vi "SMC.vi"() -> ()   [LabVIEW 2009]
doc: "This is the Superconducting Magnet Control module (SMC).\nIts job is to receive messages from the PDP, translate them into magnet commands, and send reply messages back to the PDP indicating magnet status."
uses:
  SMC Global.vi
panel:
  in  "Read\nWitness?":bool
  in  "Force Read":bool
  in  "Need to Beep":bool
  in  "Beep at Setpoint":bool=TRUE
  out "SMC Message Type":T1(ring)=enum."Ping="
  out "Magnet Entered this state at:":string
  out "Last Change":dbl format="%.2f"
  out "Update Often":bool
  out "Magnet Status":T2={"Sweep Status"=enum."To Zero", "Leads Current (A)"=0.0, "Leads Voltage (V)"=0.0, "Leads Field (T)"=0.0, "Switch Heater"=FALSE, "Setpoint (A)"=0.0, "Sweep Rate (A/min)"=0.0, "System Status"=enum."Warming Up", "Limit Status"=enum."Positive Current Limit", "Persistent Current (A)"=0.0, "Control Status"=FALSE, "Persistent Field (T)"=0.0} {"Leads Field (T)" format="%.2f"; "Persistent Field (T)" format="%.3f"; "Persistent Current (A)" format="%.3f"; "Setpoint (A)" format="%.3f"; "Leads Voltage (V)" format="%.2f"; "Sweep Rate (A/min)" format="%.2f"; "Leads Current (A)" format="%.3f"}
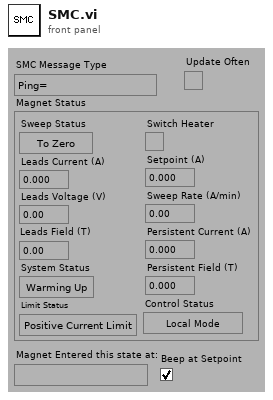
[diagram p1: front panel]
types:
  T1 = enum16{"Bad Message", "DoNothing", "Read=", "GenEvent=", "MagStatus=", "Control", "Setpoint=", "Setrate=", "Heater=", "Ping=", "Stop", "Beep"}
  T2 = cluster{"Sweep Status":enum16{"Hold", "To Setpoint", "To Zero", "Clamped"}, "Leads Current (A)":dbl, "Leads Voltage (V)":dbl, "Leads Field (T)":dbl, "Switch Heater":bool, "Setpoint (A)":dbl, "Sweep Rate (A/min)":dbl, "System Status":enum16{"Normal", "Quenched", "Over Heated", "Warming Up"}, "Limit Status":enum16{"Normal", "Positive Voltage Limit", "Negative Voltage Limit", "Negative Current Limit", "Positive Current Limit"}, "Persistent Current (A)":dbl, "Control Status":bool, "Persistent Field (T)":dbl}
  T3 = enum16{"Hold", "To Setpoint", "To Zero", "Clamped"}
  T4 = enum16{"Normal", "Quenched", "Over Heated", "Warming Up"}
  T5 = enum16{"Normal", "Positive Voltage Limit", "Negative Voltage Limit", "Negative Current Limit", "Positive Current Limit"}
  T6 = cluster{"Sweep Status":enum16{"Hold", "To Setpoint", "To Zero", "Clamped"}, "Leads Current (A)":dbl, "Leads Field (T)":dbl, "Switch Heater":bool, "Setpoint (A)":dbl, "Sweep Rate (A/min)":dbl, "System Status":enum16{"Normal", "Quenched", "Over Heated", "Warming Up"}, "Limit Status":enum16{"Normal", "Positive Voltage Limit", "Negative Voltage Limit", "Negative Current Limit", "Positive Current Limit"}, "Persistent Current (A)":dbl, "Control Status":bool, "Persistent Field (T)":dbl}
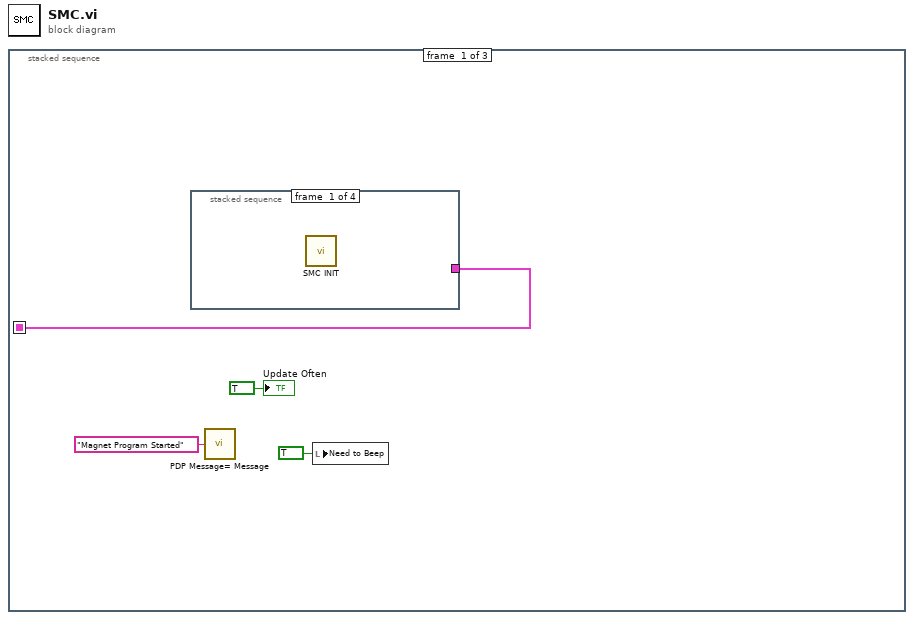
[diagram p0: block diagram]
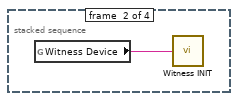
[diagram p2: hidden frame]
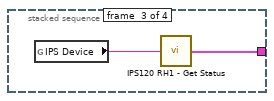
[diagram p3: hidden frame]
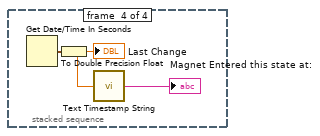
[diagram p4: hidden frame]
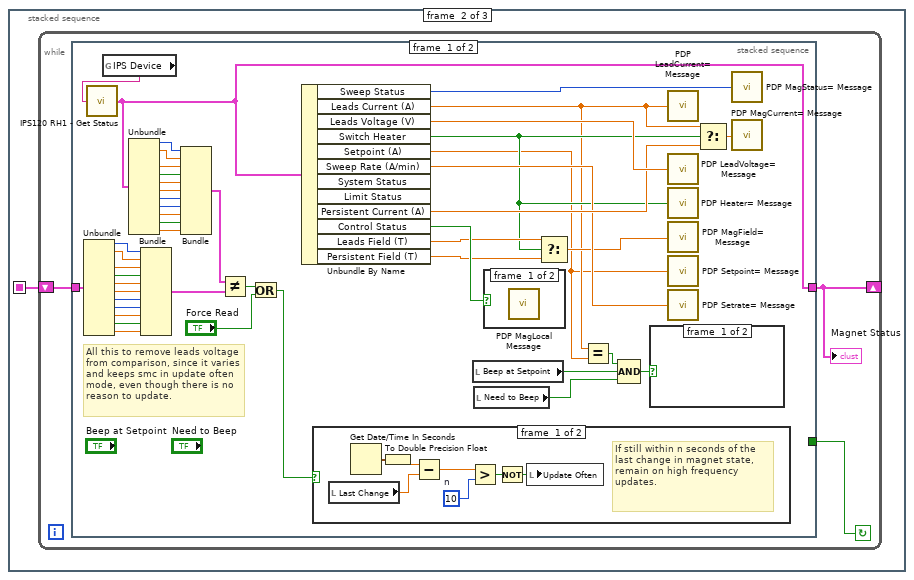
[diagram p5: hidden frame]
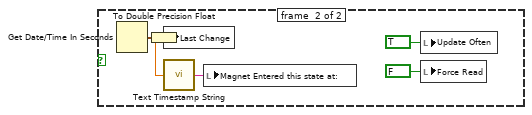
[diagram p6: hidden frame]
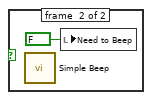
[diagram p7: hidden frame]
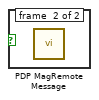
[diagram p8: hidden frame]
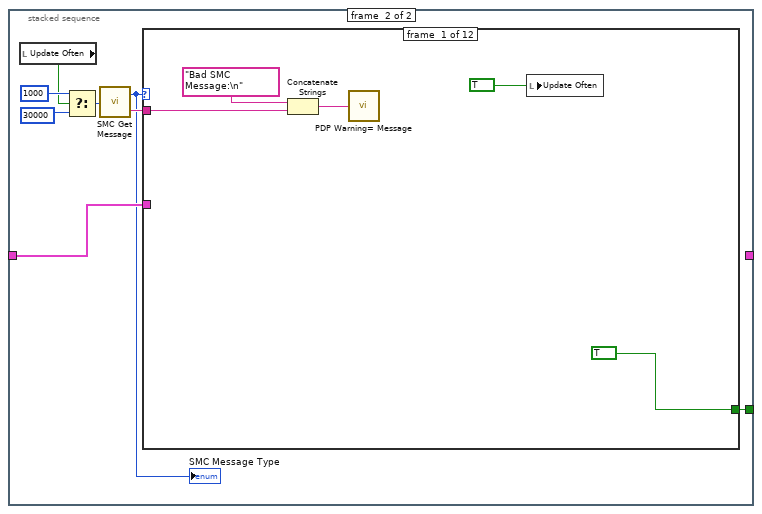
[diagram p9: hidden frame]
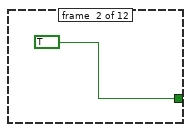
[diagram p10: hidden frame]
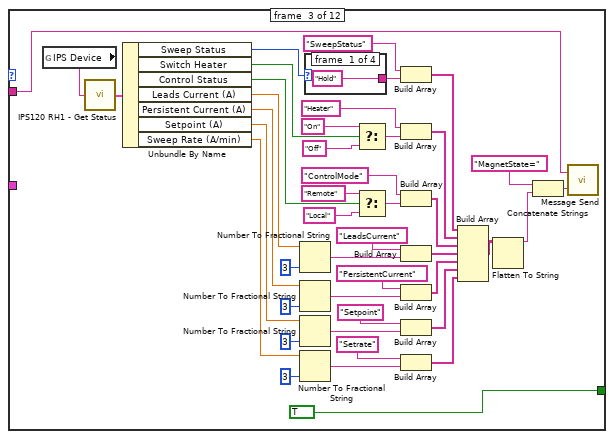
[diagram p11: hidden frame]
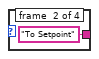
[diagram p12: hidden frame]
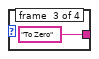
[diagram p13: hidden frame]
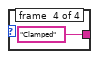
[diagram p14: hidden frame]
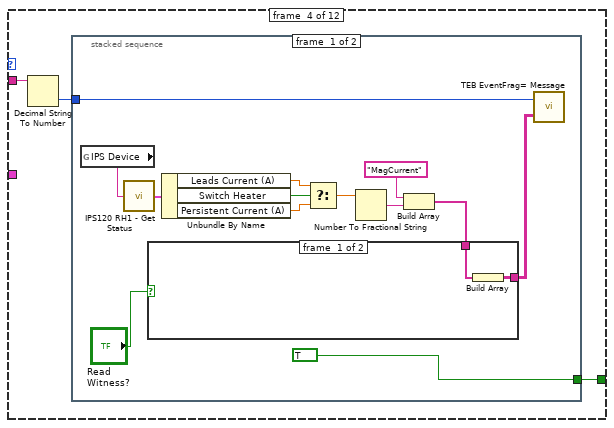
[diagram p15: hidden frame]
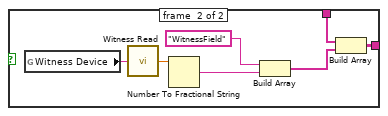
[diagram p16: hidden frame]
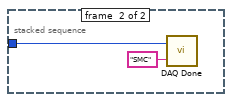
[diagram p17: hidden frame]
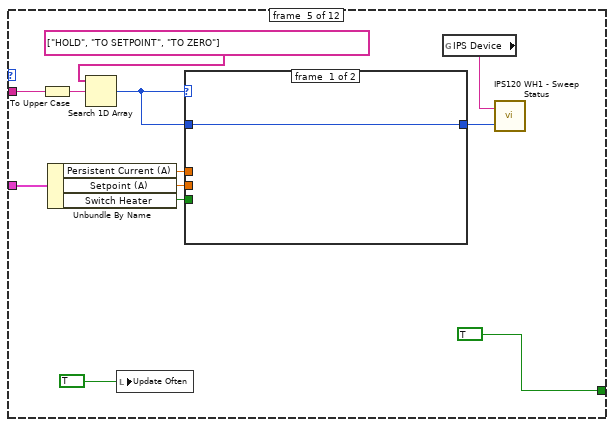
[diagram p18: hidden frame]
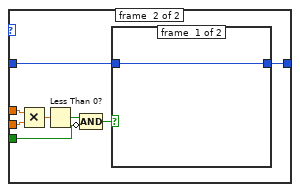
[diagram p19: hidden frame]
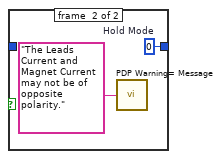
[diagram p20: hidden frame]
diagram:
  n1 = stacked-sequence {
    seq-local: [w4 _ _] -> [_ w11 _]
    frame #0 {
      n2 = stacked-sequence {
        tunnel: [_ _ w7 _] -> w4
        frame #0 {
          n3 = call "SMC INIT.vi"() -> ()  [unwired: 1 in]
        }
        frame #1 {
          n4 = global read "SMC Global.vi" "Witness Device"() -> (w5:string)
          n5 = call "Witness INIT.vi"("address string"=w5) -> ()
        }
        frame #2 {
          n6 = global read "SMC Global.vi" "IPS Device"() -> (w6:string)
          n7 = call "IPS120 RH1 - Get Status.vi"("GPIB Address"=w6) -> ("Magnet Status"=w7:T2)
        }
        frame #3 {
          n8 = Get Date/Time In Seconds() -> (seconds since 1Jan1904=w8:timestamp)
          n9 = To Double Precision Float(number=w8) -> (double precision float=w10:dbl)
          "Last Change" <- w10
          n10 = call "Text Timestamp String.vi"("Seconds"=w10) -> ("Timestamp String"=→"Magnet Entered this state at:":string)
        }
      }
      n11 = call "PDP Message= Message.vi"("Message"="Magnet Program Started") -> ()
      n12 = local write "Need to Beep"(TRUE ("Need to Beep")) -> ()
      "Update Often" <- TRUE ("Update Often")
    }
    frame #1 {
      n13 = while {
        shift-left: w11 -> [w13]
        shift-right: [w12] -> _
        stop <- w14 continue-if-true
        n14 = stacked-sequence {
          tunnel: [_ w80] -> w14
          tunnel: w13 -> [w59 w76]
          tunnel: [w45 _] -> w12
          frame #0 {
            # "All this to remove leads voltage from comparison, since it varies and keeps smc in update often mode, even though there is no \nreason to update."
            n15 = Unbundle(w59) -> ("Sweep Status"=w58:T3, "Leads Current (A)"=w57:dbl, "Leads Field (T)"=w56:dbl, "Switch Heater"=w55:bool, "Setpoint (A)"=w54:dbl, "Sweep Rate (A/min)"=w53:dbl, "System Status"=w52:T4, "Limit Status"=w51:T5, "Persistent Current (A)"=w42:dbl, "Control Status"=w41:bool, "Persistent Field (T)"=w40:dbl)  [unwired: 1 out]
            n16 = global read "SMC Global.vi" "IPS Device"() -> (w60:string)
            n17 = call "IPS120 RH1 - Get Status.vi"("GPIB Address"=w60) -> ("Magnet Status"=w45:T2)
            n18 = Unbundle(w45) -> ("Sweep Status"=w34:T3, "Leads Current (A)"=w35:dbl, "Leads Field (T)"=w36:dbl, "Switch Heater"=w37:bool, "Setpoint (A)"=w38:dbl, "Sweep Rate (A/min)"=w39:dbl, "System Status"=w50:T4, "Limit Status"=w49:T5, "Persistent Current (A)"=w48:dbl, "Control Status"=w47:bool, "Persistent Field (T)"=w46:dbl)  [unwired: 1 out]
            n19 = Bundle("Sweep Status"=w58, "Leads Current (A)"=w57, "Leads Field (T)"=w56, "Switch Heater"=w55, "Setpoint (A)"=w54, "Sweep Rate (A/min)"=w53, "System Status"=w52, "Limit Status"=w51, "Persistent Current (A)"=w42, "Control Status"=w41, "Persistent Field (T)"=w40) -> (w43:T6)  [unwired: 1 in]
            n20 = Bundle("Sweep Status"=w34, "Leads Current (A)"=w35, "Leads Field (T)"=w36, "Switch Heater"=w37, "Setpoint (A)"=w38, "Sweep Rate (A/min)"=w39, "System Status"=w50, "Limit Status"=w49, "Persistent Current (A)"=w48, "Control Status"=w47, "Persistent Field (T)"=w46) -> (w44:T6)  [unwired: 1 in]
            n21 = Not Equal?(x=w44, y=w43) -> (x != y?=w32:bool)
            n22 = Or(x=w32, y="Force Read") -> (x .or. y?=w15:bool)
            n23 = Unbundle By Name(w45) -> ("Sweep Status"=w31:T3, "Leads Current (A)"=w21:dbl, "Leads Voltage (V)"=w30:dbl, "Switch Heater"=w23:bool, "Setpoint (A)"=w20:dbl, "Sweep Rate (A/min)"=w27:dbl, "Persistent Current (A)"=w29:dbl, "Control Status"=w26:bool, "Leads Field (T)"=w25:dbl, "Persistent Field (T)"=w24:dbl)  [unwired: 2 out]
            n24 = case shown="False" w15 {
              frame #0 {
                w64 = 10  # n
                # "If still within n seconds of the last change in magnet state, remain on high frequency updates."
                n25 = local read "Last Change"() -> (w63:dbl)
                n26 = Get Date/Time In Seconds() -> (seconds since 1Jan1904=w61:timestamp)
                n27 = To Double Precision Float(number=w61) -> (double precision float=w62:dbl)
                n28 = Subtract(x=w62, y=w63) -> (x-y=w65:dbl)
                n29 = Greater?(x=w65, y=w64) -> (0:w66:bool)
                n30 = Not(x=w66) -> (.not. x?=w67:bool)
                n31 = local write "Update Often"(w67) -> ()
              }
              frame #1 {
                n32 = Get Date/Time In Seconds() -> (seconds since 1Jan1904=w68:timestamp)
                n33 = To Double Precision Float(number=w68) -> (double precision float=w71:dbl)
                n34 = local write "Last Change"(w71) -> ()
                n35 = call "Text Timestamp String.vi"("Seconds"=w71) -> ("Timestamp String"=w72:string)
                n36 = local write "Magnet Entered this state at:"(w72) -> ()
                n37 = local write "Update Often"(TRUE ("Update Often")) -> ()
                n38 = local write "Force Read"(FALSE ("Force Read")) -> ()
              }
            }
            n39 = local read "Beep at Setpoint"() -> (w18:bool)
            n40 = local read "Need to Beep"() -> (w17:bool)
            n41 = case shown="False" w26 {
              frame #0 {
                n42 = call "PDP MagLocal Message.vi"() -> ()  [unwired: 1 in]
              }
              frame #1 {
                n43 = call "PDP MagRemote Message.vi"() -> ()  [unwired: 1 in]
              }
            }
            n44 = Select(t=w25, s=w23, f=w24) -> (s? t:f=w22:dbl)
            n45 = Equal?(x=w21, y=w20) -> (x = y?=w19:bool)
            n46 = Compound Arithmetic op=AND(w19, w18, w17) -> (w16:bool)
            n47 = case shown="True" w16 {
              frame #0 {
              }
              frame #1 {
                n48 = call "Simple Beep.vi"() -> ()  [unwired: 1 in]
                n49 = local write "Need to Beep"(FALSE) -> ()
              }
            }
            n50 = call "PDP LeadCurrent= Message.vi"("Lead Current"=w21) -> ()
            n51 = call "PDP LeadVoltage= Message.vi"("Lead Voltage"=w30) -> ()
            n52 = call "PDP Heater= Message.vi"("Setrate"=w23) -> ()
            n53 = call "PDP MagField= Message.vi"("Mag Field"=w22) -> ()
            n54 = call "PDP Setpoint= Message.vi"("Setpoint"=w20) -> ()
            n55 = call "PDP Setrate= Message.vi"("Setrate"=w27) -> ()
            n56 = Select(t=w21, s=w23, f=w29) -> (s? t:f=w28:dbl)
            n57 = call "PDP MagStatus= Message.vi"("Mag Status"=w31) -> ()
            n58 = call "PDP MagCurrent= Message.vi"("Mag Current"=w28) -> ()
          }
          frame #1 {
            n59 = local read "Update Often"() -> (w74:bool)
            n60 = Select(t=1000, s=w74, f=30000) -> (s? t:f=w79:i32)
            n61 = call "SMC Get Message.vi"("Timeout (ms)"=w79) -> ("SMC Message Type"=w75:T1, "Text"=w81:string)
            "SMC Message Type" <- w75
            n62 = case shown="\"Heater=\"" w75 {
              tunnel: w81 -> [w86 _ w91 w137 w173 _ w195 w200 w204 w248 _ _]
              tunnel: [TRUE TRUE TRUE w138 TRUE TRUE TRUE TRUE TRUE TRUE FALSE TRUE] -> w80
              tunnel: w76 -> [_ _ _ _ w166 w190 _ _ _ _ _ _]
              frame #0 {
                n63 = Concatenate Strings("Bad SMC Message:\n", w86) -> (w84:string)
                n64 = call "PDP Warning= Message.vi"("Message"=w84) -> ()
                n65 = local write "Update Often"(TRUE) -> ()
              }
              frame #1 {
              }
              frame #2 {
                n66 = global read "SMC Global.vi" "IPS Device"() -> (w130:string)
                n67 = call "IPS120 RH1 - Get Status.vi"("GPIB Address"=w130) -> ("Magnet Status"=w129:T2)
                n68 = Unbundle By Name(w129) -> ("Sweep Status"=w109:T3, "Switch Heater"=w110:bool, "Control Status"=w106:bool, "Leads Current (A)"=w121:dbl, "Persistent Current (A)"=w122:dbl, "Setpoint (A)"=w123:dbl, "Sweep Rate (A/min)"=w124:dbl)
                n69 = Number To Fractional String(number=w121, precision (6)=i16 3) -> (F-format string=w120:string)  [unwired: 2 in]
                n70 = Number To Fractional String(number=w122, precision (6)=i16 3) -> (F-format string=w118:string)  [unwired: 2 in]
                n71 = Number To Fractional String(number=w123, precision (6)=i16 3) -> (F-format string=w117:string)  [unwired: 2 in]
                n72 = Number To Fractional String(number=w124, precision (6)=i16 3) -> (F-format string=w116:string)  [unwired: 2 in]
                n73 = case shown="\"Hold\"" w109 {
                  tunnel: ["Hold" "To Setpoint" "To Zero" "Clamped"] -> w101
                  frame #0 {
                  }
                  frame #1 {
                  }
                  frame #2 {
                  }
                  frame #3 {
                  }
                }
                n74 = Select(t="On", s=w110, f="Off") -> (s? t:f=w104:string)
                n75 = Select(t="Remote", s=w106, f="Local") -> (s? t:f=w105:string)
                n76 = Build Array("SweepStatus", w101) -> (w95:string[])
                n77 = Build Array("Heater", w104) -> (w94:string[])
                n78 = Build Array("ControlMode", w105) -> (w93:string[])
                n79 = Build Array("LeadsCurrent", w120) -> (w96:string[])
                n80 = Build Array("PersistentCurrent", w118) -> (w97:string[])
                n81 = Build Array("Setpoint", w117) -> (w98:string[])
                n82 = Build Array("Setrate", w116) -> (w99:string[])
                n83 = Build Array(w95, w94, w93, w96, w97, w98, w99) -> (w92:string[][])
                n84 = Flatten To String(anything=w92) -> (data string=w89:string)  [unwired: 3 in, 2 out]
                n85 = Concatenate Strings("MagnetState=" ("Substring"), w89) -> (w90:string)
                n86 = call "Message Send.vi"("Message"=w90, "Destination"=w91) -> ()
              }
              frame #3 {
                n87 = Decimal String To Number(string=w137) -> (number=w136:i32)  [unwired: 2 in, 1 out]
                n88 = stacked-sequence {
                  tunnel: [TRUE _] -> w138
                  tunnel: w136 -> [w150 w162]
                  frame #0 {
                    n89 = global read "SMC Global.vi" "IPS Device"() -> (w144:string)
                    n90 = call "IPS120 RH1 - Get Status.vi"("GPIB Address"=w144) -> ("Magnet Status"=w149:T2)
                    n91 = Unbundle By Name(w149) -> ("Leads Current (A)"=w141:dbl, "Switch Heater"=w142:bool, "Persistent Current (A)"=w140:dbl)
                    n92 = Select(t=w141, s=w142, f=w140) -> (s? t:f=w139:dbl)
                    n93 = Number To Fractional String(number=w139) -> (F-format string=w145:string)  [unwired: 3 in]
                    n94 = Build Array("MagCurrent", w145) -> (w147:string[])
                    n95 = case shown="True" "Read\nWitness?" {
                      tunnel: w147 -> [w153 w160]
                      tunnel: [w152 w159] -> w146
                      frame #0 {
                        n96 = Build Array(w153) -> (w152:string[][])
                      }
                      frame #1 {
                        n97 = global read "SMC Global.vi" "Witness Device"() -> (w154:string)
                        n98 = call "Witness Read.vi"("address string"=w154) -> ("Field"=w155:dbl)
                        n99 = Number To Fractional String(number=w155) -> (F-format string=w158:string)  [unwired: 3 in]
                        n100 = Build Array("WitnessField", w158) -> (w156:string[])
                        n101 = Build Array(w160, w156) -> (w159:string[][])
                      }
                    }
                    n102 = call "TEB EventFrag= Message.vi"("Event Fragment(s)"=w146, "Event Number"=w150) -> ()
                  }
                  frame #1 {
                    n103 = call "DAQ Done.vi"("Module Name"="SMC", "Event Number"=w162) -> ()
                  }
                }
              }
              frame #4 {
                n104 = To Upper Case(1:w173) -> (0:w172:string)
                n105 = Unbundle By Name(w166) -> ("Persistent Current (A)"=w165:dbl, "Setpoint (A)"=w164:dbl, "Switch Heater"=w163:bool)
                n106 = Search 1D Array(1D array=string[] ["HOLD", "TO SETPOINT", "TO ZERO"], element=w172) -> (index of element=w168:i32)  [unwired: 1 in]
                n107 = local write "Update Often"(TRUE) -> ()
                n108 = case shown="1.., Default" w168 {
                  tunnel: w168 -> [w175 w180]
                  tunnel: w165 -> [_ w183]
                  tunnel: w164 -> [_ w182]
                  tunnel: [w175 w179] -> w167
                  tunnel: w163 -> [_ w177]
                  frame #0 {
                  }
                  frame #1 {
                    n109 = Multiply(x=w183, y=w182) -> (x*y=w181:dbl)
                    n110 = Less Than 0?(x=w181) -> (x < 0?=w178:bool)
                    n111 = Compound Arithmetic op=AND(w178, invert w177) -> (w176:bool)
                    n112 = case shown="True" w176 {
                      tunnel: w180 -> [w184 _]
                      tunnel: [w184 w186] -> w179
                      frame #0 {
                      }
                      frame #1 {
                        w186 = 0  # Hold Mode
                        n113 = call "PDP Warning= Message.vi"("Message"="The Leads Current and Magnet Current may not be of opposite polarity.") -> ()
                      }
                    }
                  }
                }
                n114 = global read "SMC Global.vi" "IPS Device"() -> (w171:string)
                n115 = call "IPS120 WH1 - Sweep Status.vi"("Sweep Status"=w167, "GPIB Address"=w171) -> ()
              }
              frame #5 {
                n116 = global read "SMC Global.vi" "IPS Device"() -> (w187:string)
                n117 = Unbundle By Name(w190) -> ("Control Status"=w189:bool)
                n118 = Not(x=w189) -> (.not. x?=w188:bool)
                n119 = call "IPS120 WH4 - Remote Mode.vi"("Remote Mode"=w188, "GPIB Address"=w187) -> ()
              }
              frame #6 {
                w192 = TRUE
                n120 = Fract/Exp String To Number(string=w195) -> (number=w194:dbl)  [unwired: 3 in, 1 out]
                n121 = global read "SMC Global.vi" "IPS Device"() -> (w193:string)
                n122 = call "IPS120 WH2 - Write Setpoint.vi"("Setpoint"=w194, "GPIB Address"=w193) -> ()
                n123 = local write "Update Often"(w192) -> ()
                n124 = local write "Need to Beep"(w192) -> ()
              }
              frame #7 {
                n125 = Fract/Exp String To Number(string=w200) -> (number=w199:dbl)  [unwired: 3 in, 1 out]
                n126 = global read "SMC Global.vi" "IPS Device"() -> (w198:string)
                n127 = call "IPS120 WH3 - Write Setrate.vi"("Setrate"=w199, "GPIB Address"=w198) -> ()
                n128 = local write "Update Often"(TRUE) -> ()
              }
              frame #8 {
                n129 = To Upper Case(1:w204) -> (0:w202:string)
                n130 = global read "SMC Global.vi" "IPS Device"() -> (w203:string)
                n131 = case shown="\"ON\"" w202 {
                  tunnel: w203 -> [w207 w217 w232 w239]
                  frame #0 {
                    n132 = call "IPS120 RH1 - Get Status.vi"("GPIB Address"=w207) -> ("Magnet Status"=w206:T2)
                    n133 = stacked-sequence {
                      tunnel: w207 -> [w210 _ _]
                      tunnel: w206 -> [_ w212 _]
                      frame #0 {
                        n134 = call "IPS120 WH0 - Send Command.vi"("Command String"="H0", "GPIB Address"=w210) -> ()  [unwired: 1 out]
                      }
                      frame #1 {
                        # "If heater was on, wait 30 sec for it to go off."
                        n135 = Unbundle By Name(w212) -> ("Switch Heater"=w211:bool)
                        n136 = case shown="True" w211 {
                          frame #0 {
                          }
                          frame #1 {
                            n137 = stacked-sequence {
                              frame #0 {
                                n138 = call "PDP HeaterDelay= Message.vi"("Setrate"=i8 30 ("Heater Delay (sec)")) -> ()
                              }
                              frame #1 {
                                n139 = Wait (ms)(milliseconds to wait=u32 30000) -> ()  [unwired: 1 out]
                              }
                            }
                          }
                        }
                      }
                      frame #2 {
                        n140 = call "PDP Heater= Message.vi"("Setrate"=FALSE ("Switch Heater")) -> ()
                      }
                    }
                    n141 = local write "Update Often"(TRUE) -> ()
                  }
                  frame #1 {
                    n142 = call "IPS120 RH1 - Get Status.vi"("GPIB Address"=w217) -> ("Magnet Status"=w224:T2)
                    n143 = Unbundle By Name(w224) -> ("Sweep Status"=w222:T3, "Leads Current (A)"=w221:dbl, "Persistent Current (A)"=w220:dbl)
                    n144 = Equal?(x=T3."Hold" ("Sweep Status"), y=w222) -> (x = y?=w216:bool)
                    n145 = Equal?(x=w221, y=w220) -> (x = y?=w218:bool)
                    n146 = Compound Arithmetic op=AND(w216, w218) -> (w219:bool)
                    n147 = case shown="True" w219 {
                      tunnel: w218 -> [w228 _]
                      tunnel: w217 -> [_ _]
                      frame #0 {
                        n148 = Select(t="The Magnet Power Supply needs to be in Hold Mode.", s=w228, f="The Magnet Leads do not match the current in the magnet.") -> (s? t:f=w225:string)
                        n149 = call "PDP Warning= Message.vi"("Message"=w225) -> ()
                      }
                      frame #1 {
                        n150 = call "Message Send.vi"("Message"="HeaterDialog", "Destination"="PDP") -> ()
                      }
                    }
                  }
                  frame #2 {
                    n151 = stacked-sequence {
                      tunnel: w232 -> [w234 _ _ _]
                      frame #0 {
                        n152 = call "IPS120 WH0 - Send Command.vi"("Command String"="H1", "GPIB Address"=w234) -> ()  [unwired: 1 out]
                      }
                      frame #1 {
                        n153 = call "PDP HeaterDelay= Message.vi"("Setrate"=i8 30 ("Heater Delay (sec)")) -> ()
                      }
                      frame #2 {
                        n154 = Wait (ms)(milliseconds to wait=u32 30000) -> ()  [unwired: 1 out]
                      }
                      frame #3 {
                        n155 = call "PDP Heater= Message.vi"("Setrate"=TRUE ("Switch Heater")) -> ()
                      }
                    }
                    n156 = local write "Update Often"(TRUE) -> ()
                  }
                  frame #3 {
                    n157 = stacked-sequence {
                      tunnel: w239 -> [w241 _ _ _]
                      frame #0 {
                        n158 = call "IPS120 WH0 - Send Command.vi"("Command String"="H1", "GPIB Address"=w241) -> ()  [unwired: 1 out]
                      }
                      frame #1 {
                        n159 = call "PDP HeaterDelay= Message.vi"("Setrate"=i8 30 ("Heater Delay (sec)")) -> ()
                      }
                      frame #2 {
                        n160 = Wait (ms)(milliseconds to wait=u32 30000) -> ()  [unwired: 1 out]
                      }
                      frame #3 {
                        n161 = call "PDP Heater= Message.vi"("Setrate"=TRUE ("Switch Heater")) -> ()
                      }
                    }
                    n162 = local write "Update Often"(TRUE) -> ()
                  }
                }
              }
              frame #9 {
                n163 = Get Date/Time In Seconds() -> (seconds since 1Jan1904=w245:timestamp)
                n164 = To Double Precision Float(number=w245) -> (double precision float=w250:dbl)
                n165 = Format Into String(format string="PingResponse=SMC,%.0f", w250) -> (resulting string=w251:string)  [unwired: 2 in, 1 out]
                n166 = call "Message Send.vi"("Message"=w251, "Destination"=w248) -> ()
                n167 = local write "Update Often"(TRUE ("Update Often")) -> ()
              }
              frame #10 {
              }
              frame #11 {
                n168 = call <vilib>:"Beep.vi"() -> ()  [unwired: 12 in]
              }
            }
          }
        }
        "Magnet Status" <- w12
      }
    }
    frame #2 {
    }
  }
